vi "Prac.vi"() -> ()   [LabVIEW 2017]
panel:
  in  "stop":bool
  out "Gauge":dbl(knob) scale=0.0..10.0
  out "Gauge 1":dbl(knob) scale=0.0..10.0
  out "Difference Graph 2":dynamicdata(graph)
  out "Sum Graph":dynamicdata(graph)
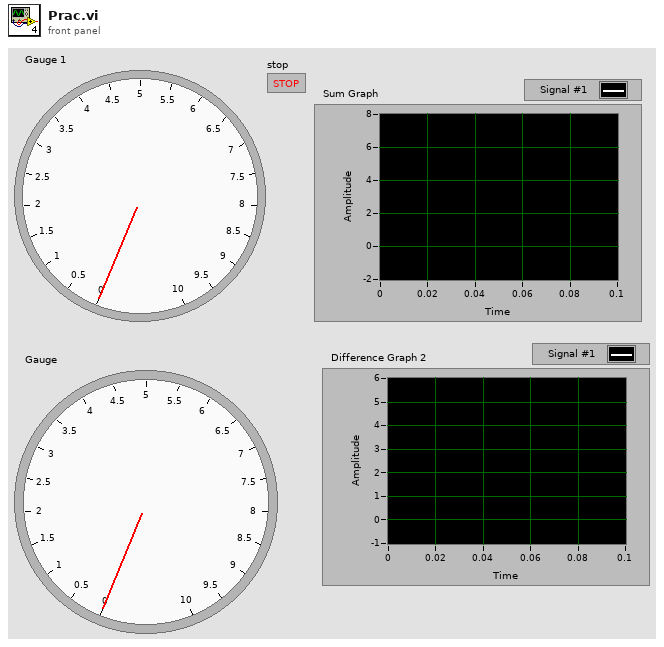
[diagram p1: front panel]
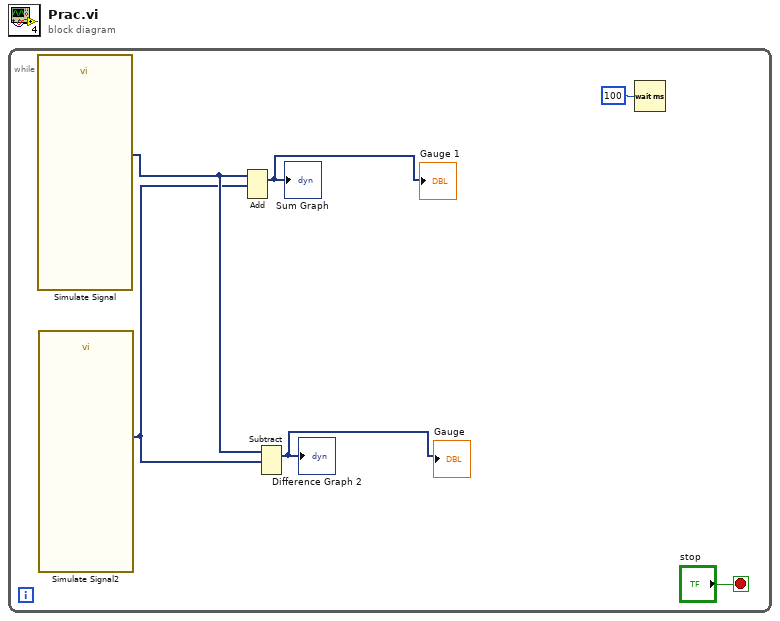
[diagram p0: block diagram]
diagram:
  n1 = while {
    stop <- "stop" stop-if-true
    n2 = call "Simulate Signal"() -> ("Signal #1"=w6:dynamicdata)  [unwired: 14 in, 1 out]
    n3 = call "Simulate Signal2"() -> ("Signal #2"=w5:dynamicdata)  [unwired: 14 in, 1 out]
    n4 = Add(1:w5, 2:w6) -> (0:→"Sum Graph" →"Gauge 1":dynamicdata)  [unwired: 1 in, 1 out]
    n5 = Subtract(1:w5, 2:w6) -> (0:→"Difference Graph 2" →"Gauge":dynamicdata)  [unwired: 1 in, 1 out]
    n6 = Wait (ms)(milliseconds to wait=u32 100) -> ()  [unwired: 1 out]
  }
